vi "QCA - DUT Commit Memory.vi"(0 "TCP Network Connection in":refnum<k5>, 1 "Commit Type":T1="otp", 5 "Write Calibration":bool=TRUE, 7 "Write PCIE":bool=TRUE, 9 "Set Command":string[](array[string])=["set ssid=3232", "set svid=168C"], 11 "error in":errorcluster={"status"=FALSE, "code"=373003, "source"="Property Node (arg 1) in niBASIC - RFSA - Waveform - Measure.vi->Calibrate NART DUT.vi->Calibrate NART DUT Example.vi->WLAN - QCA - Test Flow Control_DUT1.vi->WLAN Two Site Example_Remote PC.vi <ERR>\nOne or more channels has an ADC overload.\n\nADC overrange detected on the following channels:\nI overrange: Yes\nQ overrange: Yes"}, 12 "MAC Address":string) -> (4 "TCP Network Connection out":refnum<k5>, 15 "error out":errorcluster={"status"=FALSE, "code"=373003, "source"="Property Node (arg 1) in niBASIC - RFSA - Waveform - Measure.vi->Calibrate NART DUT.vi->Calibrate NART DUT Example.vi->WLAN - QCA - Test Flow Control_DUT1.vi->WLAN Two Site Example_Remote PC.vi <ERR>\nOne or more channels has an ADC overload.\n\nADC overrange detected on the following channels:\nI overrange: Yes\nQ overrange: Yes"})   [LabVIEW 2012]
uses:
  Controls/Commit Type.ctl
  Controls/QCA NART Response Type.ctl
  Controls/QCA NART Response SubType.ctl
  System SubVIs/Global_NB1 NB2 Ready to Go.vi
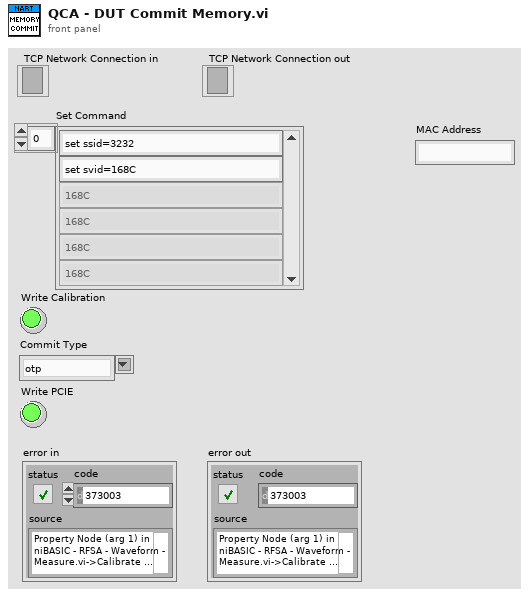
[diagram p1: front panel]
types:
  T1 = typedef "Commit Type.ctl" = string
  T2 = typedef "QCA NART Response SubType.ctl" = enum16{"NONE", "OK", "ON", "OFF", "BEGIN", "DONE"}
  T3 = typedef "QCA NART Response Type.ctl" = enum16{"DEBUG", "CONTROL", "INFO", "WARNING", "ERROR", "NONE"}
  T4 = typedef "Ctl_ART_Version.ctl" = enum16{"138", "147"}
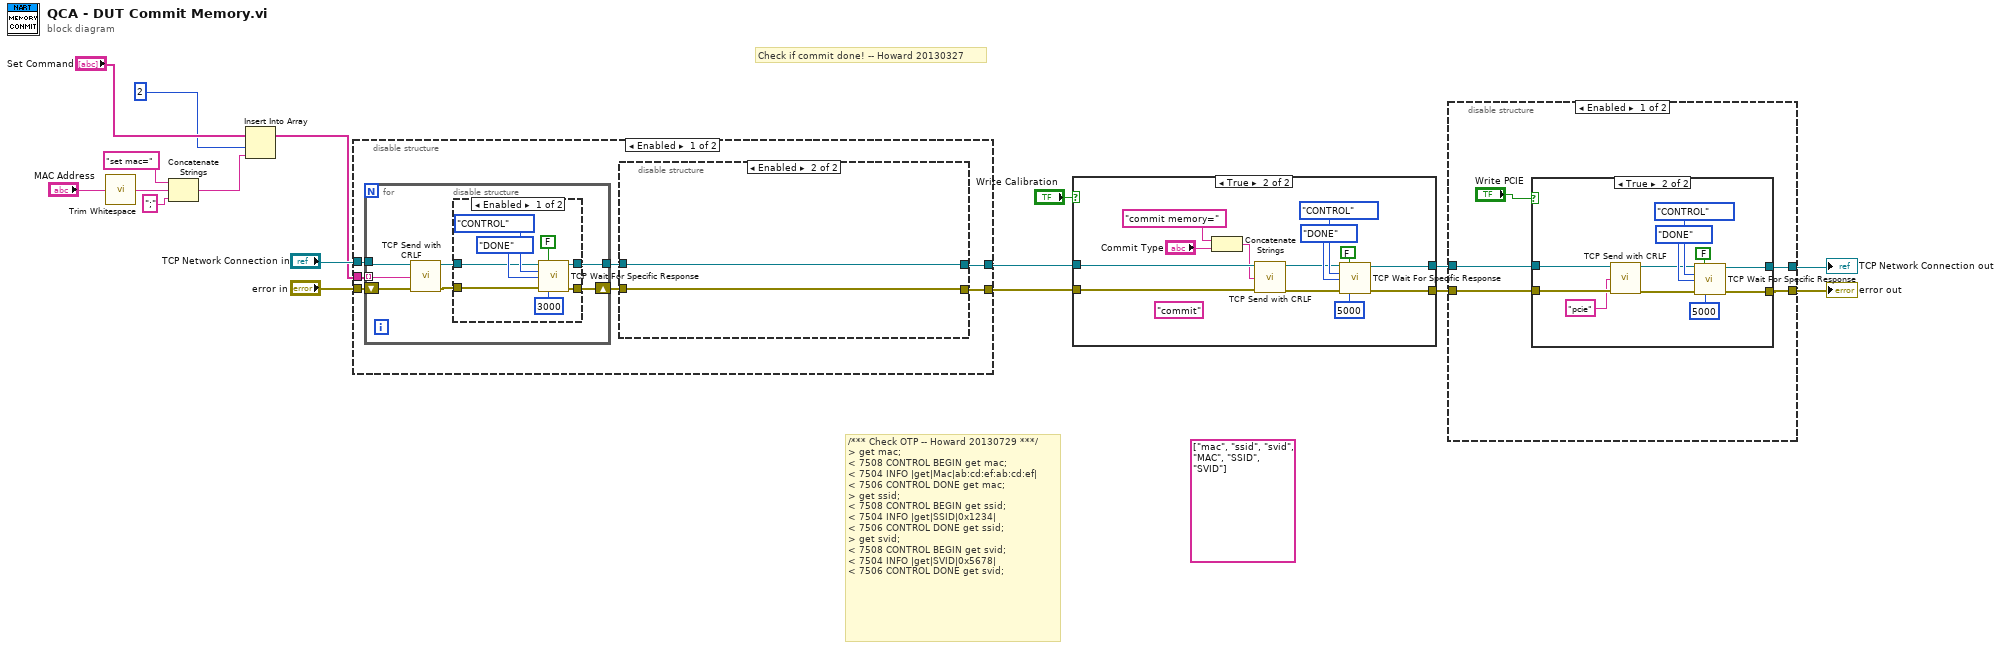
[diagram p0: block diagram]
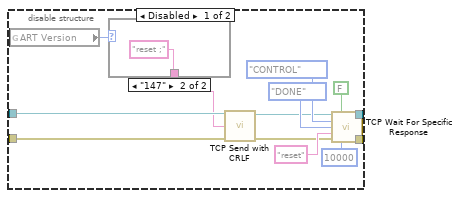
[diagram p4: hidden frame]
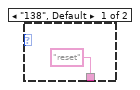
[diagram p5: hidden frame]
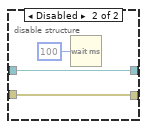
[diagram p6: hidden frame]
diagram:
  (unwired) string[] ["mac", "ssid", "svid", "MAC", "SSID", "SVID"]
  # "/*** Check OTP -- Howard 20130729 ***/\n> get mac;\n< 7508 CONTROL BEGIN get mac;\n< 7504 INFO |get|Mac|ab:cd:ef:ab:cd:ef|\n< 7506 CONTROL DONE get mac;\n> get ssid;\n< 7508 CONTROL BEGIN get ssid;\n< 7504 INFO |get|SSID|0x1234|\n< 7506 CONTROL DONE get ssid;\n> get svid;\n< 7508 CONTROL BEGIN get svid;\n< 7504 INFO |get|SVID|0x5678|\n< 7506 CONTROL DONE get svid;"
  # "Check if commit done! -- Howard 20130327"
  n1 = call <vilib>:"Trim Whitespace.vi"("string"="MAC Address") -> ("trimmed string"=w7:string)  [unwired: 1 in]
  n2 = Concatenate Strings("set mac=" ("string"), w7, ";" ("string")) -> (w2:string)
  n3 = Insert Into Array(array="Set Command", index=2, new element=w2) -> (w1:string[])
  n4 = disable-structure shown="Enabled" {
    disable-tunnel: w1 -> [w24 _]
    disable-tunnel: "TCP Network Connection in" -> [w21 w61]
    disable-tunnel: "error in" -> [w20 w60]
    disable-tunnel: [w19 w61] -> w15
    disable-tunnel: [w18 w60] -> w14
    frame Enabled {
      n5 = for {
        tunnel: [w45] -> w23
        tunnel: w21 -> [w48]
        tunnel: w24 -> [w42] mode=indexing
        shift-right: [w46] -> w22
        shift-left: w20 -> [w47]
        n6 = call "TCP Send with CRLF.vi"("CART TCP Connection"=w48, "data in"=w42, "error IO"=w47) -> ("CART TCP Connection Out"=w44:refnum<k5>, "error out"=w43:errorcluster)  [unwired: 11 in]
        n7 = disable-structure shown="Enabled" {
          disable-tunnel: [w52 w58] -> w46
          disable-tunnel: [w51 w59] -> w45
          disable-tunnel: w44 -> [w50 w59]
          disable-tunnel: w43 -> [w49 w58]
          frame Enabled {
            n8 = call "TCP Wait For Specific Response.vi"("TCP Connection In"=w50, "Next response (t)"=FALSE, "Expected Type"=QCA_NART_Response_Type."CONTROL", "Expected Subtype (none)"=QCA_NART_Response_SubType."DONE", "error in"=w49, "Timeout (250 ms)"=3000) -> ("TCP Connection Out"=w51:refnum<k5>, "error out"=w52:errorcluster)  [unwired: 6 in, 2 out]
          }
          frame Disabled {
            n9 = Wait (ms)(milliseconds to wait=u32 100) -> ()  [unwired: 1 out]
          }
        }
      }
      n10 = disable-structure shown="Enabled" {
        disable-tunnel: w23 -> [w30 w41]
        disable-tunnel: w22 -> [w29 w40]
        disable-tunnel: [w28 w41] -> w19
        disable-tunnel: [w27 w40] -> w18
        frame Disabled {
          n11 = global read "Global_NB1 NB2 Ready to Go.vi" "ART Version"() -> (w26:T4)
          n12 = case shown="\"147\"" w26 {
            tunnel: ["reset" ("data in") "reset ;"] -> w25
            frame "138", Default {
            }
            frame "147" {
            }
          }
          n13 = call "TCP Send with CRLF.vi"("CART TCP Connection"=w30, "data in"=w25, "error IO"=w29) -> ("CART TCP Connection Out"=w31:refnum<k5>, "error out"=w32:errorcluster)  [unwired: 11 in]
          n14 = call "TCP Wait For Specific Response.vi"("TCP Connection In"=w31, "Next response (t)"=FALSE, "Expected Type"=QCA_NART_Response_Type."CONTROL", "Expected Subtype (none)"=QCA_NART_Response_SubType."DONE", "Expected Message Start (\"\":any)"="reset" ("Expected Message Start (\"\":any)"), "error in"=w32, "Timeout (250 ms)"=10000) -> ("TCP Connection Out"=w28:refnum<k5>, "error out"=w27:errorcluster)  [unwired: 5 in, 2 out]
        }
        frame Enabled {
        }
      }
    }
    frame Disabled {
    }
  }
  n15 = case shown="True" "Write Calibration" {
    tunnel: w15 -> [w63 w70]
    tunnel: w14 -> [w62 w69]
    tunnel: [w63 w66] -> w11
    tunnel: [w62 w65] -> w12
    frame False {
    }
    frame True {
      (unwired) "commit"
      n16 = Concatenate Strings("commit memory=", "Commit Type") -> (w64:string)
      n17 = call "TCP Send with CRLF.vi"("CART TCP Connection"=w70, "data in"=w64, "error IO"=w69) -> ("CART TCP Connection Out"=w68:refnum<k5>, "error out"=w67:errorcluster)  [unwired: 11 in]
      n18 = call "TCP Wait For Specific Response.vi"("TCP Connection In"=w68, "Next response (t)"=FALSE, "Expected Type"=QCA_NART_Response_Type."CONTROL", "Expected Subtype (none)"=QCA_NART_Response_SubType."DONE", "error in"=w67, "Timeout (250 ms)"=5000 ("Timeout (100ms)")) -> ("TCP Connection Out"=w66:refnum<k5>, "error out"=w65:errorcluster)  [unwired: 6 in, 2 out]
    }
  }
  n19 = disable-structure shown="Enabled" {
    disable-tunnel: w12 -> [w81 w95]
    disable-tunnel: w11 -> [w80 w96]
    disable-tunnel: [w78 w96] -> w10
    disable-tunnel: [w77 w95] -> w9
    frame Enabled {
      n20 = case shown="True" "Write PCIE" {
        tunnel: w80 -> [w83 w90]
        tunnel: w81 -> [w82 w89]
        tunnel: [w83 w86] -> w78
        tunnel: [w82 w85] -> w77
        frame False {
        }
        frame True {
          n21 = call "TCP Send with CRLF.vi"("CART TCP Connection"=w90, "data in"="pcie", "error IO"=w89) -> ("CART TCP Connection Out"=w88:refnum<k5>, "error out"=w87:errorcluster)  [unwired: 11 in]
          n22 = call "TCP Wait For Specific Response.vi"("TCP Connection In"=w88, "Next response (t)"=FALSE, "Expected Type"=QCA_NART_Response_Type."CONTROL", "Expected Subtype (none)"=QCA_NART_Response_SubType."DONE", "error in"=w87, "Timeout (250 ms)"=5000 ("Timeout (100ms)")) -> ("TCP Connection Out"=w86:refnum<k5>, "error out"=w85:errorcluster)  [unwired: 6 in, 2 out]
        }
      }
    }
    frame Disabled {
    }
  }
  "TCP Network Connection out" <- w10
  "error out" <- w9
